vi "Daj Boze nesto.vi"() -> ()   [LabVIEW 2025]
uses:
  <vilib>/ptbypt/NI_PtbyPt.lvlib
  UARV/Timer/Timer 2013/Control Timer.ctl
panel:
  out "PumpFlag":bool
  out "SDFlag":bool
  out "error out":errorcluster
  in  "error in (no error)":errorcluster
  in  "Center":bool
  in  "Left":bool
  in  "Right":bool
  in  "Emergency off":bool
  in  "Off":bool
  in  "On":bool
  out "Stanje":string
  out "RightLED":bool
  out "LeftLED":bool
  out "CenterLED":bool
  out "Fault":bool
  out "On/Off":bool
  out "BrojacGreska":dbl
  out "Brojac":dbl
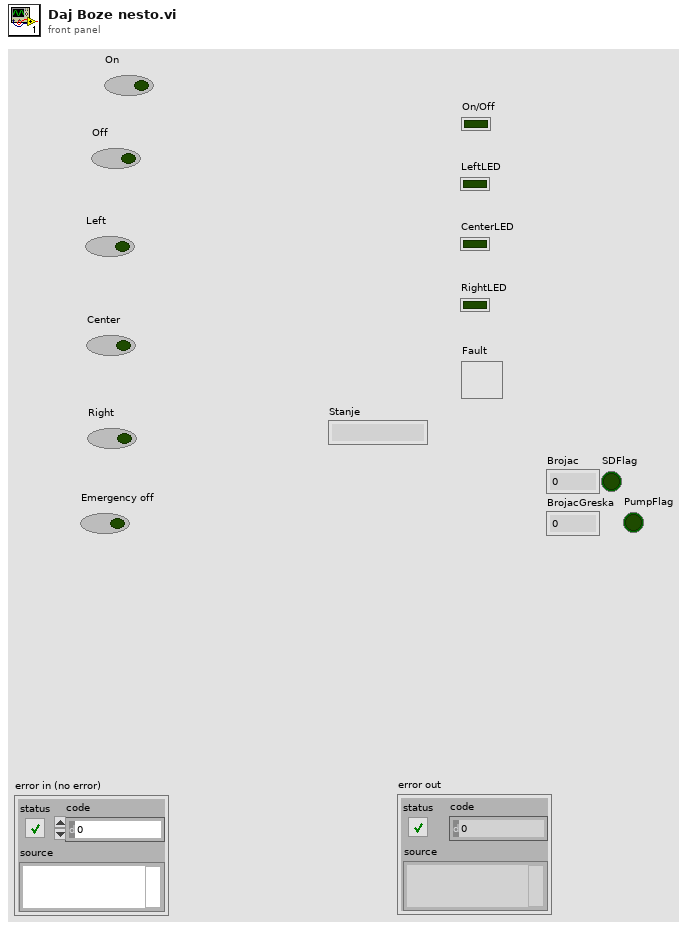
[diagram p1: front panel]
types:
  T1 = typedef "Control Timer.ctl" = enum16{"Timecheck", "Reset"}
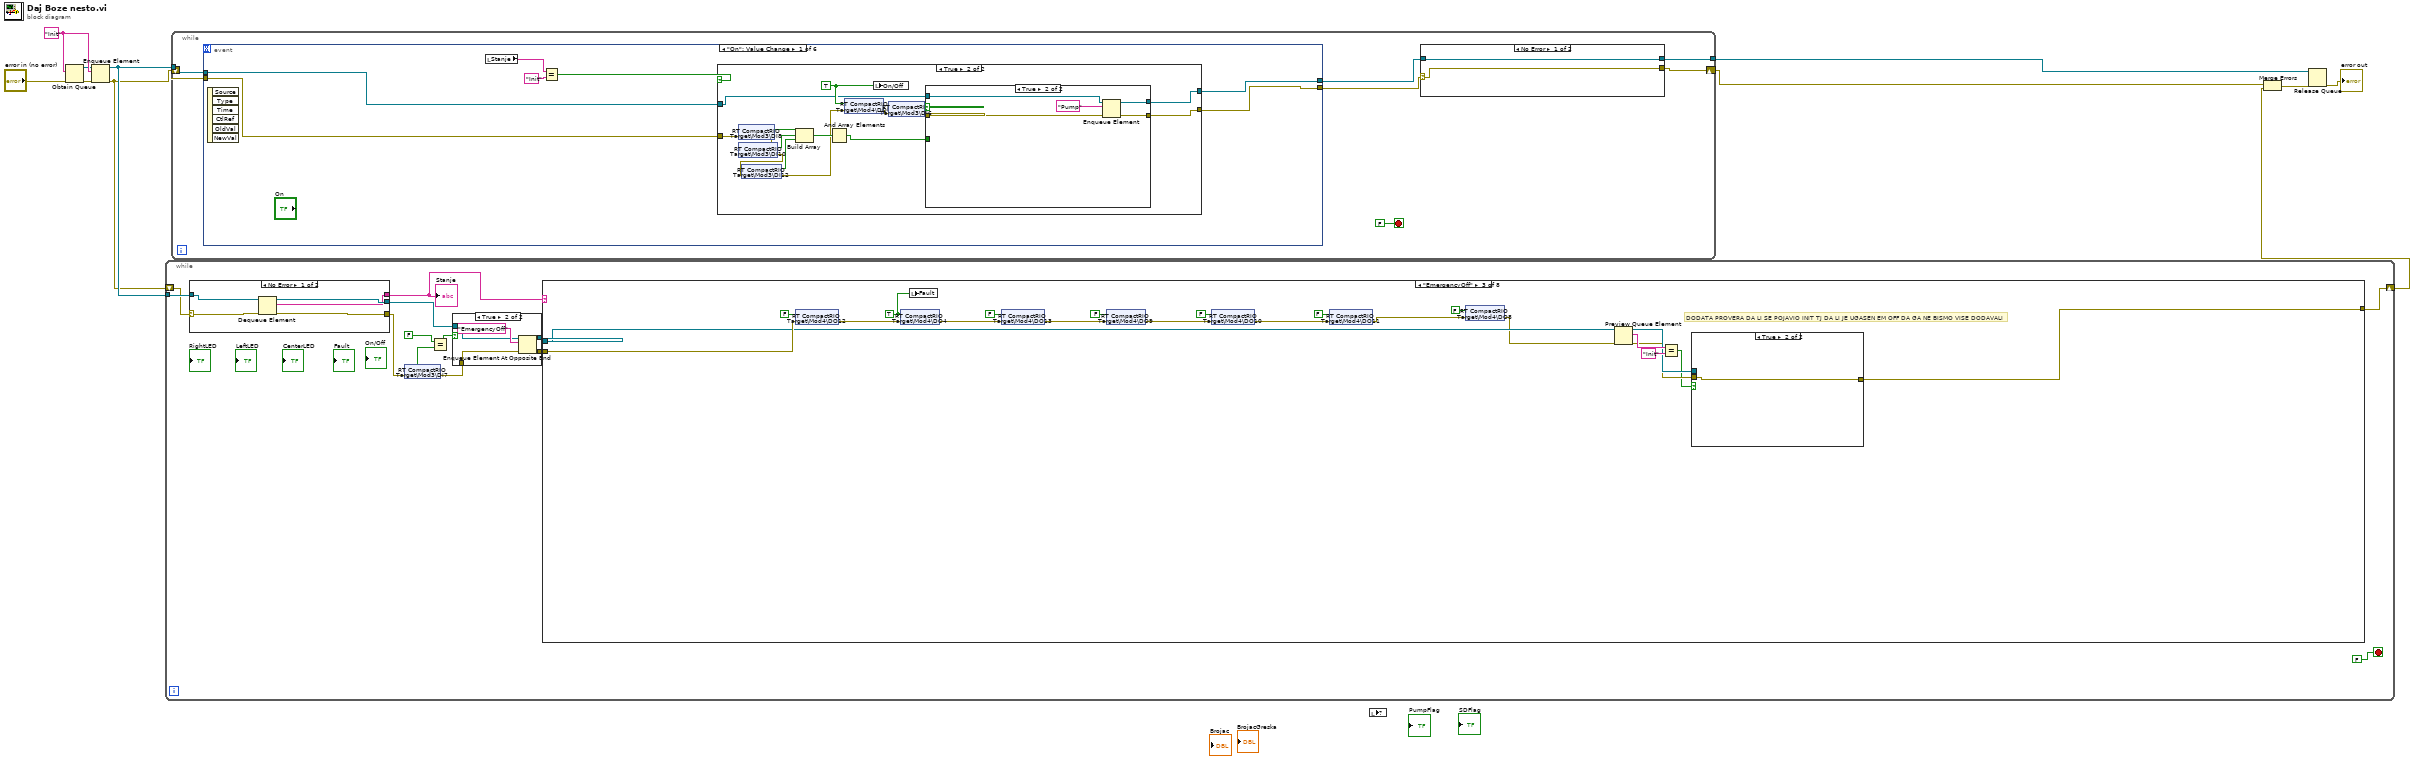
[diagram p0: block diagram]
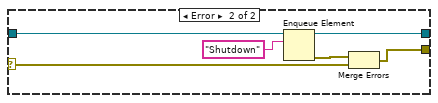
[diagram p2: hidden frame]
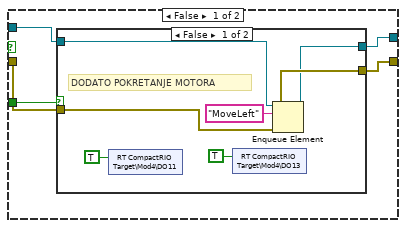
[diagram p4: hidden frame]
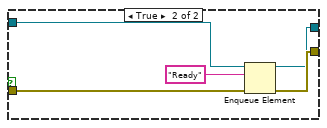
[diagram p5: hidden frame]
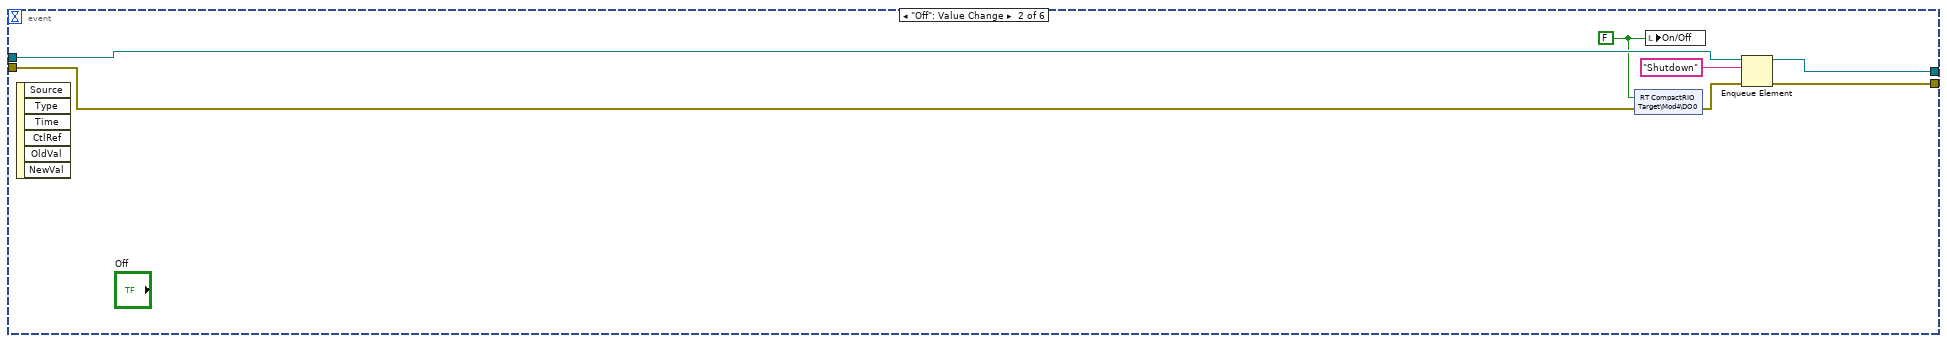
[diagram p6: hidden frame]
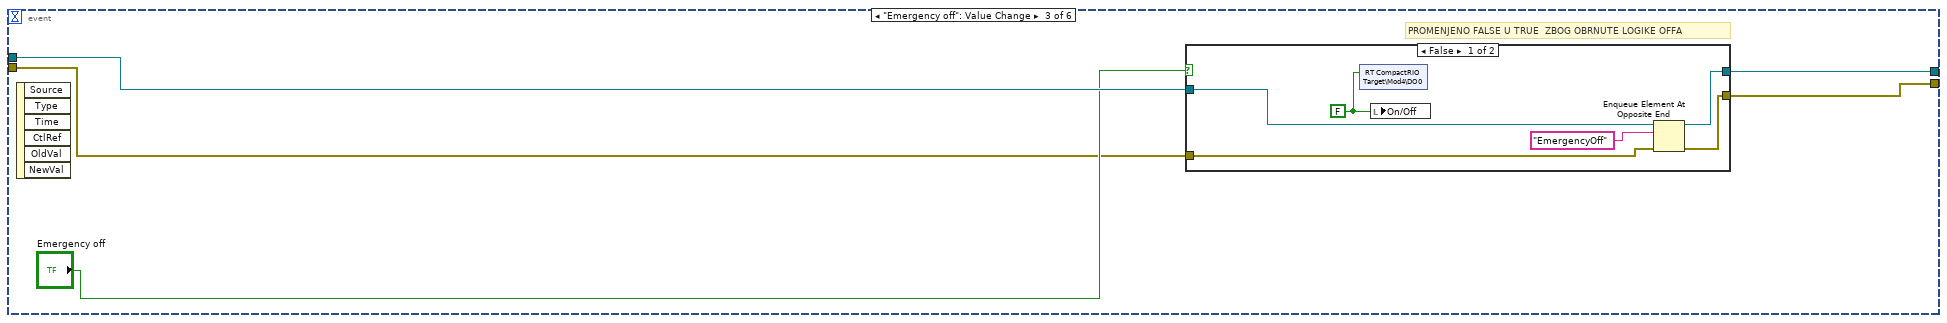
[diagram p7: hidden frame]
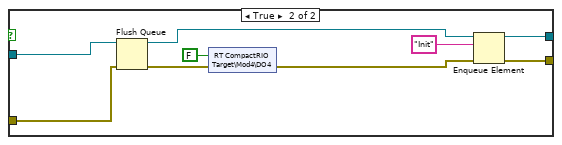
[diagram p8: hidden frame]
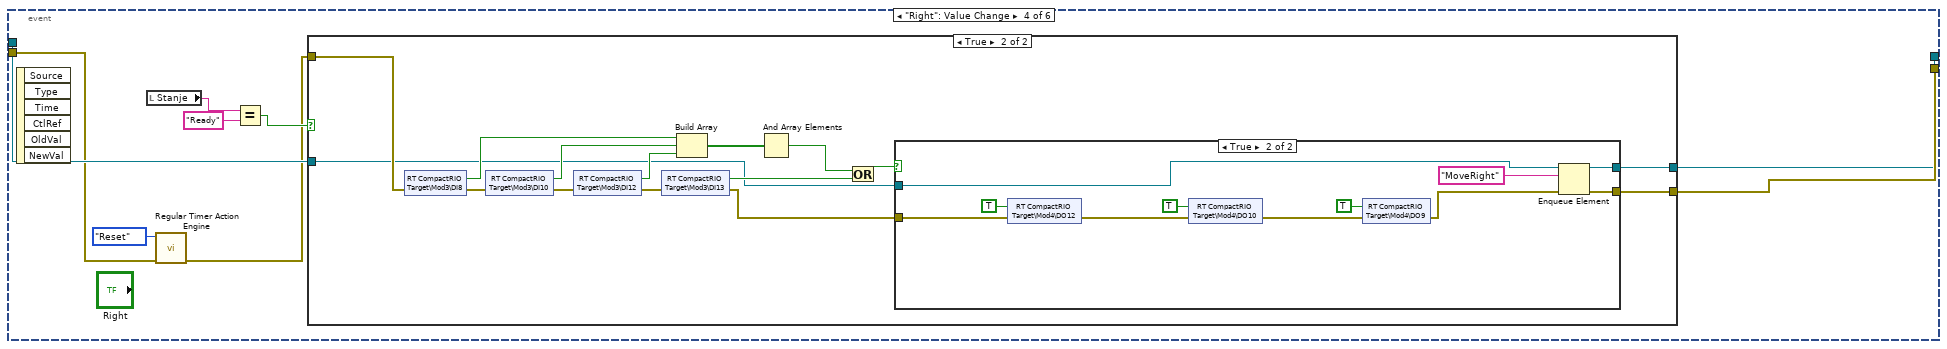
[diagram p9: hidden frame]
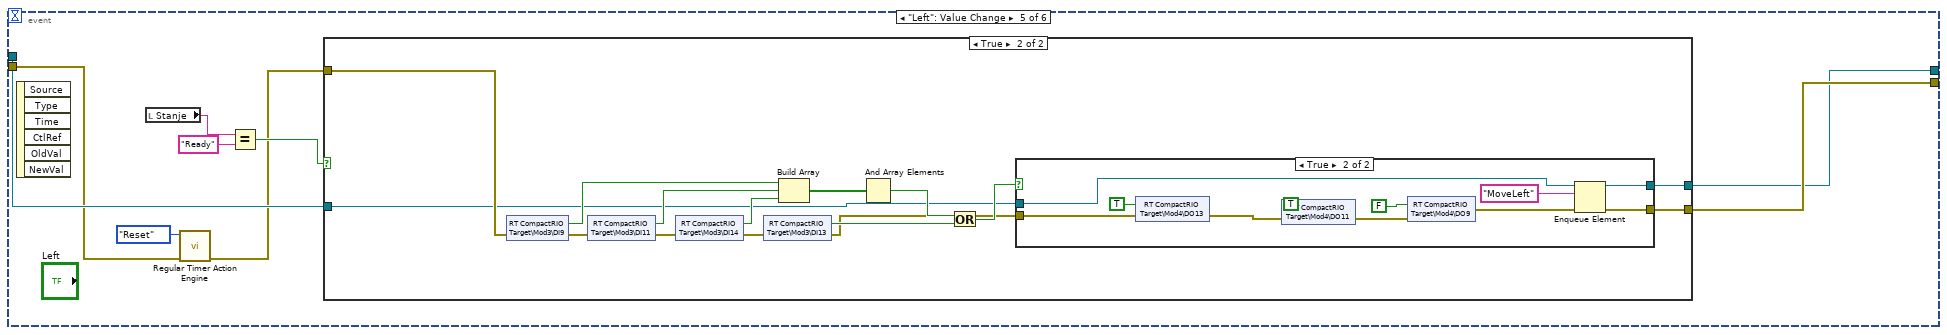
[diagram p12: hidden frame]
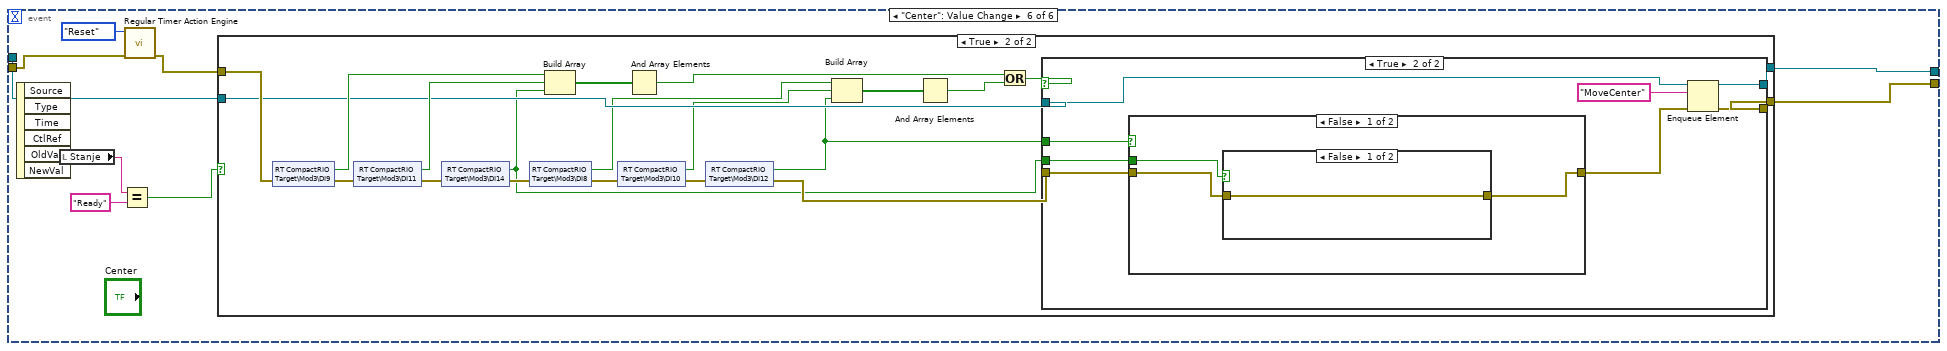
[diagram p15: hidden frame]
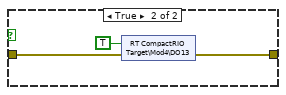
[diagram p18: hidden frame]
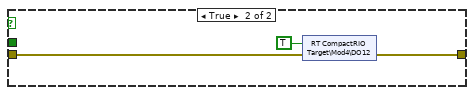
[diagram p19: hidden frame]
diagram:
  w11 = "Init"
  n1 = Obtain Queue(element data type=w11, error in (no error)="error in (no error)") -> (queue out=w9:refnum<queue>, error out=w10:errorcluster)  [unwired: 3 in, 1 out]
  n2 = Enqueue Element(queue=w9, element=w11, error in (no error)=w10) -> (queue out=w8:refnum<queue>, error out=w5:errorcluster)  [unwired: 1 in, 1 out]
  n3 = while {
    tunnel: w8 -> [w24]
    shift-right: [w12] -> w4
    shift-left: w5 -> [w13]
    stop <- FALSE stop-if-true
    n4 = case shown="No Error" w13 {
      selector: w13 -> [w567 w572]
      tunnel: w24 -> [w563 w571]
      tunnel: [w566 w570] -> w22
      tunnel: [w565 w569] -> w16
      tunnel: [w564 w568] -> w23
      frame No Error {
        n5 = Dequeue Element(queue=w563, error in (no error)=w567) -> (queue out=w565:refnum<queue>, element=w564:string, error out=w566:errorcluster)  [unwired: 1 in, 1 out]
      }
      frame Error {
        w568 = "Shutdown" ("element")
        n6 = Enqueue Element(queue=w571, element=w568, error in (no error)=w572) -> (queue out=w569:refnum<queue>, error out=w570:errorcluster)  [unwired: 1 in, 1 out]
      }
    }
    "Stanje" <- w23
    n7 = shared-variable "RT CompactRIO Target\\Mod3\\DI7"(error in=w22) -> (w21:bool, error out=w18:errorcluster)
    n8 = Equal?(x=FALSE, y=w21) -> (x = y?=w19:bool)
    n9 = case shown="True" w19 {
      tunnel: w18 -> [w26 w28]
      tunnel: [w26 w30] -> w17
      tunnel: w16 -> [w25 w27]
      tunnel: [w25 w29] -> w15
      frame False {
      }
      frame True {
        n10 = Enqueue Element At Opposite End(queue=w27, element="EmergencyOff", error in (no error)=w28) -> (queue out=w29:refnum<queue>, error out=w30:errorcluster)  [unwired: 1 in, 1 out]
      }
    }
    n11 = case shown="\"EmergencyOff\"" w23 {
      selector: w23 -> [_ _ _ _ _ _ _ w556]
      tunnel: [w43 w82 w96 w125 w148 w287 w427 w557] -> w12
      tunnel: w17 -> [w38 w86 w104 w123 w142 w281 w421 w554]
      tunnel: w15 -> [_ w81 w103 w124 w143 w282 w422 w555]
      frame "Init", Default {
        # "DOADATA REINIICILIZACIJA NOVIH PROMENLJIVIH"
        n12 = shared-variable "RT CompactRIO Target\\Mod4\\DO0"(FALSE ("DO0"), error in=w38) -> (error out=w37:errorcluster)
        n13 = shared-variable "RT CompactRIO Target\\Mod3\\DI12"(error in=w37) -> (w72:bool, error out=w70:errorcluster)
        n14 = shared-variable "RT CompactRIO Target\\Mod3\\DI10"(error in=w70) -> (w73:bool, error out=w69:errorcluster)
        n15 = shared-variable "RT CompactRIO Target\\Mod3\\DI8"(error in=w69) -> (w74:bool, error out=w59:errorcluster)
        n16 = Build Array(w74, w73, w72) -> (w71:bool[])
        n17 = And Array Elements(Boolean array=w71) -> (logical AND=w55:bool)
        n18 = local write "LeftLED"(w55) -> ()
        n19 = shared-variable "RT CompactRIO Target\\Mod4\\DO1"(w55, error in=w59) -> (error out=w58:errorcluster)
        n20 = shared-variable "RT CompactRIO Target\\Mod3\\DI14"(error in=w58) -> (w66:bool, error out=w64:errorcluster)
        n21 = shared-variable "RT CompactRIO Target\\Mod3\\DI11"(error in=w64) -> (w67:bool, error out=w63:errorcluster)
        n22 = shared-variable "RT CompactRIO Target\\Mod3\\DI9"(error in=w63) -> (w68:bool, error out=w57:errorcluster)
        n23 = Build Array(w68, w67, w66) -> (w65:bool[])
        n24 = And Array Elements(Boolean array=w65) -> (logical AND=w53:bool)
        n25 = local write "RightLED"(w53) -> ()
        n26 = shared-variable "RT CompactRIO Target\\Mod4\\DO3"(w53, error in=w57) -> (error out=w56:errorcluster)
        n27 = shared-variable "RT CompactRIO Target\\Mod3\\DI13"(error in=w56) -> (w54:bool, error out=w62:errorcluster)
        n28 = local write "Fault"(FALSE) -> ()
        n29 = local write "CenterLED"(w54) -> ()
        n30 = shared-variable "RT CompactRIO Target\\Mod4\\DO2"(w54, error in=w62) -> (error out=w51:errorcluster)
        n31 = shared-variable "RT CompactRIO Target\\Mod4\\DO4"(FALSE ("DO4"), error in=w51) -> (error out=w50:errorcluster)
        n32 = shared-variable "RT CompactRIO Target\\Mod4\\DO13"(FALSE ("DO15"), error in=w50) -> (error out=w36:errorcluster)
        n33 = shared-variable "RT CompactRIO Target\\Mod4\\DO12"(FALSE ("DO14"), error in=w36) -> (error out=w61:errorcluster)
        n34 = shared-variable "RT CompactRIO Target\\Mod4\\DO11"(FALSE ("DO13"), error in=w61) -> (error out=w42:errorcluster)
        n35 = shared-variable "RT CompactRIO Target\\Mod4\\DO8"(FALSE ("DO10"), error in=w42) -> (error out=w41:errorcluster)
        n36 = shared-variable "RT CompactRIO Target\\Mod4\\DO10"(FALSE ("DO12"), error in=w41) -> (error out=w60:errorcluster)
        n37 = shared-variable "RT CompactRIO Target\\Mod4\\DO9"(FALSE ("DO11"), error in=w60) -> (error out=w34:errorcluster)
        n38 = invoke on="SDFlag" class="Bool (strict)" method="Reinit To Default"(error in=w34) -> (error out=w33:errorcluster)  [unwired: 2 in, 2 out]
        n39 = invoke on="PumpFlag" class="Bool (strict)" method="Reinit To Default"(error in=w33) -> (error out=w32:errorcluster)  [unwired: 2 in, 2 out]
        n40 = invoke on="On/Off" class="Bool (strict)" method="Reinit To Default"(error in=w32) -> (error out=w40:errorcluster)  [unwired: 2 in, 2 out]
        n41 = invoke on="On" class="Bool (strict)" method="Reinit To Default"(error in=w40) -> (error out=w44:errorcluster)  [unwired: 2 in, 2 out]
        n42 = invoke on="Off" class="Bool (strict)" method="Reinit To Default"(error in=w44) -> (error out=w48:errorcluster)  [unwired: 2 in, 2 out]
        n43 = invoke on="Emergency off" class="Bool (strict)" method="Reinit To Default"(error in=w48) -> (error out=w47:errorcluster)  [unwired: 2 in, 2 out]
        n44 = invoke on="Right" class="Bool (strict)" method="Reinit To Default"(error in=w47) -> (error out=w46:errorcluster)  [unwired: 2 in, 2 out]
        n45 = invoke on="Left" class="Bool (strict)" method="Reinit To Default"(error in=w46) -> (error out=w45:errorcluster)  [unwired: 2 in, 2 out]
        n46 = invoke on="Center" class="Bool (strict)" method="Reinit To Default"(error in=w45) -> (error out=w43:errorcluster)  [unwired: 2 in, 2 out]
      }
      frame "Shutdown" {
        n47 = shared-variable "RT CompactRIO Target\\Mod4\\DO8"(FALSE ("DO8"), error in=w86) -> (error out=w85:errorcluster)
        n48 = shared-variable "RT CompactRIO Target\\Mod4\\DO9"(FALSE ("DO11"), error in=w85) -> (error out=w95:errorcluster)
        n49 = shared-variable "RT CompactRIO Target\\Mod4\\DO10"(FALSE ("DO12"), error in=w95) -> (error out=w87:errorcluster)
        n50 = shared-variable "RT CompactRIO Target\\Mod4\\DO11"(FALSE ("DO13"), error in=w87) -> (error out=w94:errorcluster)
        n51 = shared-variable "RT CompactRIO Target\\Mod4\\DO12"(FALSE ("DO14"), error in=w94) -> (error out=w93:errorcluster)
        n52 = shared-variable "RT CompactRIO Target\\Mod4\\DO13"(FALSE ("DO15"), error in=w93) -> (error out=w83:errorcluster)
        n53 = Enqueue Element(queue=w81, element="Init", error in (no error)=w83) -> (error out=w82:errorcluster)  [unwired: 1 in, 2 out]
      }
      frame "EmergencyOff" {
        w107 = TRUE ("DO4")
        # "DODATA PROVERA DA LI SE POJAVIO INIT TJ DA LI JE UGASEN EM OFF DA GA NE BISMO VISE DODAVALI"
        n54 = shared-variable "RT CompactRIO Target\\Mod4\\DO12"(FALSE ("DO14"), error in=w104) -> (error out=w109:errorcluster)
        n55 = shared-variable "RT CompactRIO Target\\Mod4\\DO4"(w107, error in=w109) -> (error out=w108:errorcluster)
        n56 = local write "Fault"(w107) -> ()
        n57 = shared-variable "RT CompactRIO Target\\Mod4\\DO13"(FALSE ("DO15"), error in=w108) -> (error out=w111:errorcluster)
        n58 = shared-variable "RT CompactRIO Target\\Mod4\\DO9"(FALSE ("DO11"), error in=w111) -> (error out=w117:errorcluster)
        n59 = shared-variable "RT CompactRIO Target\\Mod4\\DO10"(FALSE ("DO12"), error in=w117) -> (error out=w110:errorcluster)
        n60 = shared-variable "RT CompactRIO Target\\Mod4\\DO11"(FALSE ("DO13"), error in=w110) -> (error out=w106:errorcluster)
        n61 = shared-variable "RT CompactRIO Target\\Mod4\\DO8"(FALSE ("DO8"), error in=w106) -> (error out=w100:errorcluster)
        n62 = Preview Queue Element(queue=w103, error in (no error)=w100) -> (queue out=w99:refnum<queue>, element=w102:string, error out=w98:errorcluster)  [unwired: 1 in, 1 out]
        n63 = Equal?(x=w102, y="Init") -> (x = y?=w97:bool)
        n64 = case shown="True" w97 {
          tunnel: w99 -> [w120 _]
          tunnel: w98 -> [w119 w122]
          tunnel: [w118 w122] -> w96
          frame False {
            n65 = Enqueue Element At Opposite End(queue=w120, element="EmergencyOff", error in (no error)=w119) -> (error out=w118:errorcluster)  [unwired: 1 in, 2 out]
          }
          frame True {
          }
        }
      }
      frame "Pump" {
        n66 = shared-variable "RT CompactRIO Target\\Mod3\\DI6"(error in=w123) -> (w128:bool, error out=w126:errorcluster)
        n67 = call <vilib>:"Boolean Crossing PtByPt.vi"("direction"=enum16{"either", "false-true", "true-false"}."true-false", "input"=w128) -> ("crossing"=w127:bool)  [unwired: 1 in]
        n68 = case shown="False" w127 {
          tunnel: w126 -> [w132 w138]
          tunnel: [w135 w141] -> w125
          tunnel: w124 -> [w130 w136]
          frame False {
            n69 = shared-variable "RT CompactRIO Target\\Mod4\\DO8"(TRUE ("DO10"), error in=w132) -> (error out=w131:errorcluster)
            n70 = Enqueue Element(queue=w130, element="Pump", error in (no error)=w131) -> (error out=w135:errorcluster)  [unwired: 1 in, 2 out]
          }
          frame True {
            n71 = shared-variable "RT CompactRIO Target\\Mod4\\DO8"(FALSE ("DO10"), error in=w138) -> (error out=w137:errorcluster)
            n72 = Enqueue Element(queue=w136, element="Ready", error in (no error)=w137) -> (error out=w141:errorcluster)  [unwired: 1 in, 2 out]
          }
        }
      }
      frame "MoveRight" {
        n73 = shared-variable "RT CompactRIO Target\\Mod3\\DI6"(error in=w142) -> (w146:bool, error out=w147:errorcluster)
        n74 = call <vilib>:"Boolean Crossing PtByPt.vi"("direction"=enum16{"either", "false-true", "true-false"}."false-true", "input"=w146) -> ("crossing"=w144:bool)  [unwired: 1 in]
        n75 = case shown="False" w144 {
          tunnel: w147 -> [w178 w280]
          tunnel: [w175 w280] -> w148
          tunnel: w143 -> [w157 _]
          frame False {
            n76 = shared-variable "RT CompactRIO Target\\Mod3\\DI9"(error in=w178) -> (w182:bool, error out=w177:errorcluster)
            n77 = shared-variable "RT CompactRIO Target\\Mod3\\DI11"(error in=w177) -> (w181:bool, error out=w176:errorcluster)
            n78 = shared-variable "RT CompactRIO Target\\Mod3\\DI14"(error in=w176) -> (w180:bool, error out=w164:errorcluster)
            n79 = shared-variable "RT CompactRIO Target\\Mod3\\DI12"(error in=w164) -> (w171:bool, error out=w169:errorcluster)
            n80 = Build Array(w182, w181, w180) -> (w179:bool[])
            n81 = shared-variable "RT CompactRIO Target\\Mod3\\DI10"(error in=w169) -> (w172:bool, error out=w168:errorcluster)
            n82 = And Array Elements(Boolean array=w179) -> (logical AND=w174:bool)
            n83 = shared-variable "RT CompactRIO Target\\Mod3\\DI8"(error in=w168) -> (w173:bool, error out=w167:errorcluster)
            n84 = shared-variable "RT CompactRIO Target\\Mod3\\DI13"(error in=w167) -> (w162:bool, error out=w166:errorcluster)
            n85 = Build Array(w173, w172, w171) -> (w170:bool[])
            n86 = local write "CenterLED"(w162) -> ()
            n87 = shared-variable "RT CompactRIO Target\\Mod4\\DO2"(w162, error in=w166) -> (error out=w165:errorcluster)
            n88 = And Array Elements(Boolean array=w170) -> (logical AND=w163:bool)
            n89 = shared-variable "RT CompactRIO Target\\Mod4\\DO1"(w163, error in=w165) -> (error out=w156:errorcluster)
            n90 = local write "LeftLED"(w163) -> ()
            n91 = Preview Queue Element(queue=w157, error in (no error)=w156) -> (queue out=w154:refnum<queue>, element=w150:string, error out=w155:errorcluster)  [unwired: 1 in, 1 out]
            n92 = Equal?(x=w150, y="Shutdown") -> (x = y?=w151:bool)
            n93 = case shown="True" w151 {
              tunnel: w155 -> [w183 w188]
              tunnel: w154 -> [w184 w187]
              tunnel: [w184 w186] -> w153
              tunnel: [w183 w185] -> w152
              frame False {
              }
              frame True {
                n94 = Flush Queue(queue=w187, error in (no error)=w188) -> (queue out=w186:refnum<queue>, error out=w185:errorcluster)  [unwired: 1 out]
                n95 = local write "SDFlag"(TRUE ("SDFlag")) -> ()
              }
            }
            n96 = feedback #1() -> (w161:dbl)  [unwired: 1 in]
            n97 = feedback #2() -> (w159:dbl)  [unwired: 1 in]
            n98 = case shown="True" w174 {
              tunnel: [w198 w260] -> w175
              tunnel: w161 -> [w195 _]
              tunnel: [w194 0.0] -> w160
              tunnel: w159 -> [w193 _]
              tunnel: [w192 0.0] -> w158
              tunnel: w153 -> [w190 w251]
              tunnel: w152 -> [w191 w250]
              frame False {
                n99 = call "Regular Timer Action Engine.vi"("Enum"=Control_Timer."Timecheck", "Time Target"=0.5, "error in"=w191) -> ("Status"=w204:cluster{"Running":bool, "Done":bool}, "error out"=w201:errorcluster)  [unwired: 6 in]
                n100 = Unbundle By Name(w204) -> ("Done"=w203:bool)  [unwired: 1 out]
                n101 = feedback #3() -> (w202:bool)  [unwired: 1 in]
                n102 = case shown="True" w203 {
                  tunnel: [w212 w231] -> w197
                  tunnel: w202 -> [w212 w230]
                  tunnel: w201 -> [w211 w228]
                  tunnel: [w211 w222] -> w200
                  tunnel: w193 -> [w210 w227]
                  tunnel: [w210 w223] -> w192
                  tunnel: w195 -> [w209 w221]
                  tunnel: [w209 w218] -> w194
                  tunnel: [w208 w217] -> w196
                  tunnel: w190 -> [w208 w213]
                  frame False {
                  }
                  frame True {
                    n103 = Increment(x=w227) -> (x+1=w224:dbl)
                    n104 = Increment(x=w221) -> (x+1=w216:dbl)
                    n105 = local write "Brojac"(w224) -> ()
                    n106 = local write "BrojacGreska"(w216) -> ()
                    n107 = Not(x=w230) -> (.not. x?=w231:bool)
                    n108 = Equal?(x=w216, y=30.0) -> (x = y?=w219:bool)
                    n109 = Equal?(x=4.0, y=w224) -> (x = y?=w226:bool)
                    n110 = call "Regular Timer Action Engine.vi"("Enum"=Control_Timer."Reset", "error in"=w228) -> ("error out"=w215:errorcluster)  [unwired: 7 in, 1 out]
                    n111 = case shown="True" w219 {
                      tunnel: [w234 0.0] -> w218
                      tunnel: w216 -> [w234 _]
                      tunnel: [w232 w238] -> w217
                      tunnel: w215 -> [w233 w237]
                      tunnel: [w233 w236] -> w214
                      tunnel: w213 -> [w232 w235]
                      frame False {
                      }
                      frame True {
                        n112 = Flush Queue(queue=w235, error in (no error)=w237) -> (queue out=w240:refnum<queue>, error out=w241:errorcluster)  [unwired: 1 out]
                        n113 = Enqueue Element At Opposite End(queue=w240, element="EmergencyOff", error in (no error)=w241) -> (queue out=w238:refnum<queue>, error out=w236:errorcluster)  [unwired: 1 in, 1 out]
                      }
                    }
                    n114 = case shown="True" w226 {
                      tunnel: w224 -> [w244 _]
                      tunnel: [w244 0.0] -> w223
                      tunnel: [w243 w245] -> w222
                      tunnel: w214 -> [w243 w245]
                      frame False {
                      }
                      frame True {
                        n115 = shared-variable "RT CompactRIO Target\\Mod4\\DO10"(FALSE ("DO12")) -> ()  [unwired: 1 in, 1 out]
                      }
                    }
                  }
                }
                n116 = feedback-in #3(w197) -> ()
                n117 = local write "RightLED"(w197) -> ()
                n118 = shared-variable "RT CompactRIO Target\\Mod4\\DO3"(w197, error in=w200) -> (error out=w199:errorcluster)
                n119 = Enqueue Element(queue=w196, element="MoveRight", error in (no error)=w199) -> (error out=w198:errorcluster)  [unwired: 1 in, 2 out]
              }
              frame True {
                w254 = TRUE ("DO3")
                # "DODATA OBRADA PUMP FLAGA AKO NIJE SD FLAG"
                n120 = shared-variable "RT CompactRIO Target\\Mod4\\DO12"(FALSE ("DO15"), error in=w250) -> (error out=w257:errorcluster)
                n121 = shared-variable "RT CompactRIO Target\\Mod4\\DO10"(FALSE ("DO13"), error in=w257) -> (error out=w256:errorcluster)
                n122 = local write "RightLED"(w254) -> ()
                n123 = shared-variable "RT CompactRIO Target\\Mod4\\DO3"(w254, error in=w256) -> (error out=w255:errorcluster)
                n124 = local read "SDFlag"() -> (w249:bool)
                n125 = local read "PumpFlag"() -> (w248:bool)
                n126 = case shown="False" w249 {
                  tunnel: [w264 w278] -> w260
                  tunnel: w255 -> [w263 w274]
                  tunnel: w251 -> [w262 w275]
                  tunnel: w248 -> [w261 _]
                  frame False {
                    n127 = case shown="True" w261 {
                      tunnel: [w267 w271] -> w264
                      tunnel: w263 -> [w266 w272]
                      tunnel: w262 -> [w265 w273]
                      frame False {
                        n128 = Enqueue Element(queue=w265, element="Ready", error in (no error)=w266) -> (error out=w267:errorcluster)  [unwired: 1 in, 2 out]
                      }
                      frame True {
                        n129 = local write "PumpFlag"(FALSE ("PumpFlag")) -> ()
                        n130 = Enqueue Element(queue=w273, element="Pump", error in (no error)=w272) -> (error out=w271:errorcluster)  [unwired: 1 in, 2 out]
                      }
                    }
                  }
                  frame True {
                    n131 = local write "SDFlag"(FALSE ("SDFlag")) -> ()
                    n132 = Enqueue Element(queue=w275, element="Shutdown", error in (no error)=w274) -> (error out=w278:errorcluster)  [unwired: 1 in, 2 out]
                  }
                }
              }
            }
            n133 = feedback-in #1(w160) -> ()
            n134 = feedback-in #2(w158) -> ()
          }
          frame True {
            # "DODAT FALG UMESTO POKRETANJA PUMPE ODMAH"
            n135 = local write "PumpFlag"(TRUE ("PumpFlag")) -> ()
          }
        }
      }
      frame "MoveLeft" {
        n136 = shared-variable "RT CompactRIO Target\\Mod3\\DI6"(error in=w281) -> (w286:bool, error out=w284:errorcluster)
        n137 = call <vilib>:"Boolean Crossing PtByPt.vi"("direction"=enum16{"either", "false-true", "true-false"}."false-true", "input"=w286) -> ("crossing"=w283:bool)  [unwired: 1 in]
        n138 = case shown="False" w283 {
          tunnel: w284 -> [w316 w419]
          tunnel: [w313 w419] -> w287
          tunnel: w282 -> [w289 _]
          frame False {
            n139 = shared-variable "RT CompactRIO Target\\Mod3\\DI8"(error in=w316) -> (w321:bool, error out=w315:errorcluster)
            n140 = shared-variable "RT CompactRIO Target\\Mod3\\DI10"(error in=w315) -> (w320:bool, error out=w314:errorcluster)
            n141 = shared-variable "RT CompactRIO Target\\Mod3\\DI12"(error in=w314) -> (w319:bool, error out=w308:errorcluster)
            n142 = shared-variable "RT CompactRIO Target\\Mod3\\DI14"(error in=w308) -> (w310:bool, error out=w307:errorcluster)
            n143 = Build Array(w321, w320, w319) -> (w318:bool[])
            n144 = shared-variable "RT CompactRIO Target\\Mod3\\DI11"(error in=w307) -> (w311:bool, error out=w306:errorcluster)
            n145 = And Array Elements(Boolean array=w318) -> (logical AND=w317:bool)
            n146 = shared-variable "RT CompactRIO Target\\Mod3\\DI9"(error in=w306) -> (w312:bool, error out=w305:errorcluster)
            n147 = shared-variable "RT CompactRIO Target\\Mod3\\DI13"(error in=w305) -> (w301:bool, error out=w304:errorcluster)
            n148 = Build Array(w312, w311, w310) -> (w309:bool[])
            n149 = shared-variable "RT CompactRIO Target\\Mod4\\DO2"(w301, error in=w304) -> (error out=w303:errorcluster)
            n150 = local write "CenterLED"(w301) -> ()
            n151 = And Array Elements(Boolean array=w309) -> (logical AND=w302:bool)
            n152 = local write "RightLED"(w302) -> ()
            n153 = shared-variable "RT CompactRIO Target\\Mod4\\DO3"(w302, error in=w303) -> (error out=w296:errorcluster)
            n154 = Preview Queue Element(queue=w289, error in (no error)=w296) -> (queue out=w292:refnum<queue>, element=w295:string, error out=w291:errorcluster)  [unwired: 1 in, 1 out]
            n155 = Equal?(x=w295, y="Shutdown") -> (x = y?=w293:bool)
            n156 = case shown="True" w293 {
              tunnel: w292 -> [w322 w328]
              tunnel: w291 -> [w323 w327]
              tunnel: [w323 w326] -> w290
              tunnel: [w322 w324] -> w288
              frame False {
              }
              frame True {
                n157 = Flush Queue(queue=w328, error in (no error)=w327) -> (queue out=w324:refnum<queue>, error out=w326:errorcluster)  [unwired: 1 out]
                n158 = local write "SDFlag"(TRUE ("SDFlag")) -> ()
              }
            }
            n159 = feedback #4() -> (w300:dbl)  [unwired: 1 in]
            n160 = feedback #5() -> (w298:dbl)  [unwired: 1 in]
            n161 = case shown="True" w317 {
              tunnel: w290 -> [w333 w396]
              tunnel: [w346 w400] -> w313
              tunnel: w288 -> [w336 w392]
              tunnel: w300 -> [w332 _]
              tunnel: [w331 0.0] -> w299
              tunnel: w298 -> [w330 _]
              tunnel: [w329 0.0] -> w297
              frame False {
                n162 = call "Regular Timer Action Engine.vi"("Enum"=Control_Timer."Timecheck", "Time Target"=0.5, "error in"=w333) -> ("Status"=w342:cluster{"Running":bool, "Done":bool}, "error out"=w339:errorcluster)  [unwired: 6 in]
                n163 = Unbundle By Name(w342) -> ("Done"=w341:bool)  [unwired: 1 out]
                n164 = feedback #6() -> (w340:bool)  [unwired: 1 in]
                n165 = case shown="True" w341 {
                  tunnel: [w351 w370] -> w337
                  tunnel: w340 -> [w351 w369]
                  tunnel: w339 -> [w350 w358]
                  tunnel: [w350 w367] -> w334
                  tunnel: [w349 w363] -> w329
                  tunnel: w330 -> [w349 w366]
                  tunnel: w332 -> [w348 w354]
                  tunnel: w336 -> [w347 w360]
                  tunnel: [w347 w359] -> w335
                  tunnel: [w348 w355] -> w331
                  frame False {
                  }
                  frame True {
                    n166 = Increment(x=w366) -> (x+1=w353:dbl)
                    n167 = local write "Brojac"(w353) -> ()
                    n168 = Increment(x=w354) -> (x+1=w352:dbl)
                    n169 = local write "BrojacGreska"(w352) -> ()
                    n170 = Equal?(x=w352, y=30.0) -> (x = y?=w361:bool)
                    n171 = Equal?(x=w353, y=4.0) -> (x = y?=w364:bool)
                    n172 = Not(x=w369) -> (.not. x?=w370:bool)
                    n173 = case shown="True" w364 {
                      tunnel: w353 -> [w383 _]
                      tunnel: [w383 0.0] -> w363
                      tunnel: w358 -> [w382 w385]
                      tunnel: [w382 w384] -> w357
                      frame False {
                      }
                      frame True {
                        n174 = shared-variable "RT CompactRIO Target\\Mod4\\DO11"(FALSE ("DO13"), error in=w385) -> (error out=w384:errorcluster)
                      }
                    }
                    n175 = case shown="True" w361 {
                      tunnel: w352 -> [w373 _]
                      tunnel: [w373 0.0] -> w355
                      tunnel: w360 -> [w372 w380]
                      tunnel: [w372 w378] -> w359
                      tunnel: w357 -> [w371 w377]
                      tunnel: [w371 w375] -> w356
                      frame False {
                      }
                      frame True {
                        n176 = Flush Queue(queue=w380, error in (no error)=w377) -> (queue out=w379:refnum<queue>, error out=w376:errorcluster)  [unwired: 1 out]
                        n177 = Enqueue Element At Opposite End(queue=w379, element="EmergencyOff", error in (no error)=w376) -> (queue out=w378:refnum<queue>, error out=w375:errorcluster)  [unwired: 1 in, 1 out]
                      }
                    }
                    n178 = call "Regular Timer Action Engine.vi"("Enum"=Control_Timer."Reset", "error in"=w356) -> ("error out"=w367:errorcluster)  [unwired: 7 in, 1 out]
                  }
                }
                n179 = feedback-in #6(w337) -> ()
                n180 = local write "LeftLED"(w337) -> ()
                n181 = shared-variable "RT CompactRIO Target\\Mod4\\DO1"(w337, error in=w334) -> (error out=w338:errorcluster)
                n182 = Enqueue Element(queue=w335, element="MoveLeft", error in (no error)=w338) -> (error out=w346:errorcluster)  [unwired: 1 in, 2 out]
              }
              frame True {
                w394 = TRUE ("DO1")
                # "DODATA OBRADA PUMP FLAGA AKO NIJE SD FLAG"
                n183 = local write "LeftLED"(w394) -> ()
                n184 = shared-variable "RT CompactRIO Target\\Mod4\\DO1"(w394, error in=w396) -> (error out=w395:errorcluster)
                n185 = shared-variable "RT CompactRIO Target\\Mod4\\DO13"(FALSE ("DO15"), error in=w395) -> (error out=w397:errorcluster)
                n186 = local read "SDFlag"() -> (w389:bool)
                n187 = local read "PumpFlag"() -> (w388:bool)
                n188 = shared-variable "RT CompactRIO Target\\Mod4\\DO11"(FALSE ("DO13"), error in=w397) -> (error out=w393:errorcluster)
                n189 = case shown="False" w389 {
                  tunnel: [w404 w416] -> w400
                  tunnel: w393 -> [w403 w418]
                  tunnel: w392 -> [w402 w417]
                  tunnel: w388 -> [w401 _]
                  frame False {
                    n190 = case shown="True" w401 {
                      tunnel: [w407 w411] -> w404
                      tunnel: w403 -> [w406 w413]
                      tunnel: w402 -> [w405 w412]
                      frame False {
                        n191 = Enqueue Element(queue=w405, element="Ready", error in (no error)=w406) -> (error out=w407:errorcluster)  [unwired: 1 in, 2 out]
                      }
                      frame True {
                        n192 = local write "PumpFlag"(FALSE ("PumpFlag")) -> ()
                        n193 = Enqueue Element(queue=w412, element="Pump", error in (no error)=w413) -> (error out=w411:errorcluster)  [unwired: 1 in, 2 out]
                      }
                    }
                  }
                  frame True {
                    n194 = Enqueue Element(queue=w417, element="Shutdown", error in (no error)=w418) -> (error out=w416:errorcluster)  [unwired: 1 in, 2 out]
                    n195 = local write "SDFlag"(FALSE ("SDFlag")) -> ()
                  }
                }
              }
            }
            n196 = feedback-in #4(w299) -> ()
            n197 = feedback-in #5(w297) -> ()
          }
          frame True {
            # "DODAT FALG UMESTO POKRETANJA PUMPE ODMAH"
            n198 = local write "PumpFlag"(TRUE ("PumpFlag")) -> ()
          }
        }
      }
      frame "MoveCenter" {
        n199 = shared-variable "RT CompactRIO Target\\Mod3\\DI6"(error in=w421) -> (w426:bool, error out=w423:errorcluster)
        n200 = call <vilib>:"Boolean Crossing PtByPt.vi"("direction"=enum16{"either", "false-true", "true-false"}."false-true", "input"=w426) -> ("crossing"=w424:bool)  [unwired: 1 in]
        n201 = case shown="False" w424 {
          tunnel: [w459 w541] -> w427
          tunnel: w423 -> [w445 w541]
          tunnel: w422 -> [w435 _]
          frame False {
            n202 = shared-variable "RT CompactRIO Target\\Mod3\\DI12"(error in=w445) -> (w455:bool, error out=w453:errorcluster)
            n203 = shared-variable "RT CompactRIO Target\\Mod3\\DI10"(error in=w453) -> (w456:bool, error out=w452:errorcluster)
            n204 = shared-variable "RT CompactRIO Target\\Mod3\\DI8"(error in=w452) -> (w457:bool, error out=w444:errorcluster)
            n205 = shared-variable "RT CompactRIO Target\\Mod3\\DI14"(error in=w444) -> (w449:bool, error out=w447:errorcluster)
            n206 = Build Array(w457, w456, w455) -> (w454:bool[])
            n207 = shared-variable "RT CompactRIO Target\\Mod3\\DI11"(error in=w447) -> (w450:bool, error out=w446:errorcluster)
            n208 = And Array Elements(Boolean array=w454) -> (logical AND=w439:bool)
            n209 = shared-variable "RT CompactRIO Target\\Mod3\\DI9"(error in=w446) -> (w451:bool, error out=w443:errorcluster)
            n210 = local write "LeftLED"(w439) -> ()
            n211 = shared-variable "RT CompactRIO Target\\Mod4\\DO1"(w439, error in=w443) -> (error out=w442:errorcluster)
            n212 = Build Array(w451, w450, w449) -> (w448:bool[])
            n213 = And Array Elements(Boolean array=w448) -> (logical AND=w440:bool)
            n214 = local write "RightLED"(w440) -> ()
            n215 = shared-variable "RT CompactRIO Target\\Mod4\\DO3"(w440, error in=w442) -> (error out=w441:errorcluster)
            n216 = shared-variable "RT CompactRIO Target\\Mod3\\DI13"(error in=w441) -> (w458:bool, error out=w436:errorcluster)
            n217 = Preview Queue Element(queue=w435, error in (no error)=w436) -> (queue out=w431:refnum<queue>, element=w434:string, error out=w430:errorcluster)  [unwired: 1 in, 1 out]
            n218 = Equal?(x=w434, y="Shutdown") -> (x = y?=w432:bool)
            n219 = case shown="True" w432 {
              tunnel: w431 -> [w461 w466]
              tunnel: w430 -> [w460 w465]
              tunnel: [w460 w464] -> w429
              tunnel: [w461 w462] -> w428
              frame False {
              }
              frame True {
                n220 = local write "SDFlag"(TRUE ("SDFlag")) -> ()
                n221 = Flush Queue(queue=w466, error in (no error)=w465) -> (queue out=w462:refnum<queue>, error out=w464:errorcluster)  [unwired: 1 out]
              }
            }
            n222 = feedback #7() -> (w438:dbl)  [unwired: 1 in]
            n223 = case shown="True" w458 {
              tunnel: [w474 w522] -> w459
              tunnel: w429 -> [w475 w520]
              tunnel: w428 -> [w470 w515]
              tunnel: [w468 0.0] -> w437
              tunnel: w438 -> [w467 _]
              frame False {
                n224 = call "Regular Timer Action Engine.vi"("Enum"=Control_Timer."Timecheck", "Time Target"=0.5, "error in"=w475) -> ("Status"=w479:cluster{"Running":bool, "Done":bool}, "error out"=w476:errorcluster)  [unwired: 6 in]
                n225 = Unbundle By Name(w479) -> ("Done"=w478:bool)  [unwired: 1 out]
                n226 = feedback #8() -> (w477:bool)  [unwired: 1 in]
                n227 = case shown="False" w478 {
                  tunnel: [w486 w499] -> w471
                  tunnel: w477 -> [w486 w498]
                  tunnel: w476 -> [w485 w490]
                  tunnel: [w485 w496] -> w473
                  tunnel: w470 -> [w484 w492]
                  tunnel: [w484 w491] -> w469
                  tunnel: [w483 w488] -> w468
                  tunnel: w467 -> [w483 w487]
                  frame False {
                  }
                  frame True {
                    n228 = Increment(x=w487) -> (x+1=w493:dbl)
                    n229 = local write "BrojacGreska"(w493) -> ()
                    n230 = Equal?(x=w493, y=30.0) -> (x = y?=w494:bool)
                    n231 = case shown="True" w494 {
                      tunnel: [w502 0.0] -> w488
                      tunnel: w493 -> [w502 _]
                      tunnel: w492 -> [w500 w508]
                      tunnel: [w500 w506] -> w491
                      tunnel: w490 -> [w501 w505]
                      tunnel: [w501 w503] -> w489
                      frame False {
                      }
                      frame True {
                        n232 = Flush Queue(queue=w508, error in (no error)=w505) -> (queue out=w507:refnum<queue>, error out=w504:errorcluster)  [unwired: 1 out]
                        n233 = Enqueue Element At Opposite End(queue=w507, element="EmergencyOff", error in (no error)=w504) -> (queue out=w506:refnum<queue>, error out=w503:errorcluster)  [unwired: 1 in, 1 out]
                      }
                    }
                    n234 = Not(x=w498) -> (.not. x?=w499:bool)
                    n235 = call "Regular Timer Action Engine.vi"("Enum"=Control_Timer."Reset", "error in"=w489) -> ("error out"=w496:errorcluster)  [unwired: 7 in, 1 out]
                  }
                }
                n236 = feedback-in #8(w471) -> ()
                n237 = local write "CenterLED"(w471) -> ()
                n238 = shared-variable "RT CompactRIO Target\\Mod4\\DO2"(w471, error in=w473) -> (error out=w472:errorcluster)
                n239 = Enqueue Element(queue=w469, element="MoveCenter", error in (no error)=w472) -> (error out=w474:errorcluster)  [unwired: 1 in, 2 out]
              }
              frame True {
                w516 = TRUE ("DO2")
                # "DODATA OBRADA PUMP FLAGA AKO NIJE SD FLAG"
                n240 = shared-variable "RT CompactRIO Target\\Mod4\\DO13"(FALSE ("DO15"), error in=w520) -> (error out=w519:errorcluster)
                n241 = shared-variable "RT CompactRIO Target\\Mod4\\DO12"(FALSE ("DO14"), error in=w519) -> (error out=w518:errorcluster)
                n242 = local write "CenterLED"(w516) -> ()
                n243 = shared-variable "RT CompactRIO Target\\Mod4\\DO2"(w516, error in=w518) -> (error out=w517:errorcluster)
                n244 = local read "SDFlag"() -> (w512:bool)
                n245 = local read "PumpFlag"() -> (w511:bool)
                n246 = case shown="False" w512 {
                  tunnel: [w526 w538] -> w522
                  tunnel: w517 -> [w525 w540]
                  tunnel: w515 -> [w524 w539]
                  tunnel: w511 -> [w523 _]
                  frame False {
                    n247 = case shown="True" w523 {
                      tunnel: [w529 w533] -> w526
                      tunnel: w525 -> [w528 w535]
                      tunnel: w524 -> [w527 w534]
                      frame False {
                        n248 = Enqueue Element(queue=w527, element="Ready", error in (no error)=w528) -> (error out=w529:errorcluster)  [unwired: 1 in, 2 out]
                      }
                      frame True {
                        n249 = local write "PumpFlag"(FALSE ("PumpFlag")) -> ()
                        n250 = Enqueue Element(queue=w534, element="Pump", error in (no error)=w535) -> (error out=w533:errorcluster)  [unwired: 1 in, 2 out]
                      }
                    }
                  }
                  frame True {
                    n251 = local write "SDFlag"(FALSE ("SDFlag")) -> ()
                    n252 = Enqueue Element(queue=w539, element="Shutdown", error in (no error)=w540) -> (error out=w538:errorcluster)  [unwired: 1 in, 2 out]
                  }
                }
              }
            }
            n253 = feedback-in #7(w437) -> ()
          }
          frame True {
            # "DODAT FALG UMESTO POKRETANJA PUMPE ODMAH"
            n254 = local write "PumpFlag"(TRUE ("PumpFlag")) -> ()
          }
        }
      }
      frame "Ready" {
        n255 = Preview Queue Element(queue=w555, error in (no error)=w554) -> (queue out=w553:refnum<queue>, element=w550:string, error out=w552:errorcluster)  [unwired: 1 in, 1 out]
        n256 = Equal?(x=w550, y="MoveRight") -> (x = y?=w547:bool)
        n257 = Equal?(x=w550, y="MoveLeft") -> (x = y?=w546:bool)
        n258 = Equal?(x=w550, y="MoveCenter") -> (x = y?=w544:bool)
        n259 = Or(x=w547, y=w546) -> (x .or. y?=w545:bool)
        n260 = Or(x=w545, y=w544) -> (x .or. y?=w543:bool)
        n261 = case shown="False" w543 {
          tunnel: [w561 w562] -> w557
          tunnel: w556 -> [w560 _]
          tunnel: w553 -> [w559 _]
          tunnel: w552 -> [w558 w562]
          frame False {
            n262 = Enqueue Element(queue=w559, element=w560, error in (no error)=w558) -> (error out=w561:errorcluster)  [unwired: 1 in, 2 out]
          }
          frame True {
          }
        }
      }
    }
  }
  n263 = while {
    tunnel: w8 -> [w579]
    tunnel: [w576] -> w6
    shift-right: [w574] -> w3
    shift-left: w5 -> [w573]
    stop <- FALSE stop-if-true
    n264 = event shown="[0] \"On\": Value Change" {
      selector: _ -> [_ _ _ _ _ _]
      dyn-events: _ -> [_ _ _ _ _ _]
      timeout: _ -> [_ _ _ _ _ _]
      tunnel: w579 -> [w589 w640 w646 w668 w707 w746]
      tunnel: [w594 w639 w645 w670 w709 w748] -> w578
      tunnel: [w593 w638 w644 w669 w708 w747] -> w577
      tunnel: w573 -> [w588 w635 w642 w662 w701 w740]
      event "On": Value Change {
        n265 = event-data() -> ()  [unwired: 1 in, 6 out]
        n266 = local read "Stanje"() -> (w590:string)
        n267 = Equal?(x=w590, y="Init") -> (x = y?=w591:bool)
        n268 = case shown="True" w591 {
          tunnel: [w595 w612] -> w594
          tunnel: [w596 w611] -> w593
          tunnel: w589 -> [w596 w598]
          tunnel: w588 -> [w595 w597]
          frame False {
          }
          frame True {
            w599 = TRUE
            n269 = shared-variable "RT CompactRIO Target\\Mod3\\DI8"(error in=w597) -> (w605:bool, error out=w602:errorcluster)
            n270 = shared-variable "RT CompactRIO Target\\Mod3\\DI10"(error in=w602) -> (w606:bool, error out=w601:errorcluster)
            n271 = shared-variable "RT CompactRIO Target\\Mod3\\DI12"(error in=w601) -> (w607:bool, error out=w600:errorcluster)
            n272 = Build Array(w605, w606, w607) -> (w604:bool[])
            n273 = And Array Elements(Boolean array=w604) -> (logical AND=w603:bool)
            n274 = shared-variable "RT CompactRIO Target\\Mod4\\DO0"(w599, error in=w600) -> (error out=w608:errorcluster)
            n275 = local write "On/Off"(w599) -> ()
            n276 = shared-variable "RT CompactRIO Target\\Mod3\\DI6"(error in=w608) -> (w610:bool, error out=w609:errorcluster)
            n277 = case shown="True" w610 {
              tunnel: [w617 w633] -> w612
              tunnel: [w616 w632] -> w611
              tunnel: w609 -> [w615 w631]
              tunnel: w603 -> [w614 _]
              tunnel: w598 -> [w613 w630]
              frame False {
                n278 = case shown="False" w614 {
                  tunnel: [w623 w629] -> w617
                  tunnel: [w622 w627] -> w616
                  tunnel: w615 -> [w624 w626]
                  tunnel: w613 -> [w620 w625]
                  frame False {
                    # "DODATO POKRETANJE MOTORA"
                    n279 = shared-variable "RT CompactRIO Target\\Mod4\\DO11"(TRUE ("DO11")) -> ()  [unwired: 1 in, 1 out]
                    n280 = shared-variable "RT CompactRIO Target\\Mod4\\DO13"(TRUE ("DO13")) -> ()  [unwired: 1 in, 1 out]
                    n281 = Enqueue Element(queue=w620, element="MoveLeft", error in (no error)=w624) -> (queue out=w622:refnum<queue>, error out=w623:errorcluster)  [unwired: 1 in, 1 out]
                  }
                  frame True {
                    n282 = Enqueue Element(queue=w625, element="Ready", error in (no error)=w626) -> (queue out=w627:refnum<queue>, error out=w629:errorcluster)  [unwired: 1 in, 1 out]
                  }
                }
              }
              frame True {
                n283 = Enqueue Element(queue=w630, element="Pump", error in (no error)=w631) -> (queue out=w632:refnum<queue>, error out=w633:errorcluster)  [unwired: 1 in, 1 out]
              }
            }
          }
        }
      }
      event "Off": Value Change {
        w636 = FALSE
        n284 = event-data() -> ()  [unwired: 1 in, 6 out]
        n285 = shared-variable "RT CompactRIO Target\\Mod4\\DO0"(w636, error in=w635) -> (error out=w637:errorcluster)
        n286 = local write "On/Off"(w636) -> ()
        n287 = Enqueue Element(queue=w640, element="Shutdown", error in (no error)=w637) -> (queue out=w638:refnum<queue>, error out=w639:errorcluster)  [unwired: 1 in, 1 out]
      }
      event "Emergency off": Value Change {
        # "PROMENJENO FALSE U TRUE  ZBOG OBRNUTE LOGIKE OFFA"
        n288 = event-data() -> ()  [unwired: 1 in, 6 out]
        n289 = case shown="False" "Emergency off" {
          tunnel: w646 -> [w651 w661]
          tunnel: [w650 w660] -> w645
          tunnel: [w649 w659] -> w644
          tunnel: w642 -> [w647 w653]
          frame False {
            w648 = FALSE
            n290 = shared-variable "RT CompactRIO Target\\Mod4\\DO0"(w648) -> ()  [unwired: 1 in, 1 out]
            n291 = local write "On/Off"(w648) -> ()
            n292 = Enqueue Element At Opposite End(queue=w651, element="EmergencyOff", error in (no error)=w647) -> (queue out=w649:refnum<queue>, error out=w650:errorcluster)  [unwired: 1 in, 1 out]
          }
          frame True {
            n293 = Flush Queue(queue=w661, error in (no error)=w653) -> (queue out=w658:refnum<queue>, error out=w655:errorcluster)  [unwired: 1 out]
            n294 = shared-variable "RT CompactRIO Target\\Mod4\\DO4"(FALSE ("DO4"), error in=w655) -> (error out=w654:errorcluster)
            n295 = Enqueue Element(queue=w658, element="Init", error in (no error)=w654) -> (queue out=w659:refnum<queue>, error out=w660:errorcluster)  [unwired: 1 in, 1 out]
          }
        }
      }
      event "Right": Value Change {
        n296 = event-data() -> ()  [unwired: 1 in, 6 out]
        n297 = local read "Stanje"() -> (w667:string)
        n298 = call "Regular Timer Action Engine.vi"("Enum"=Control_Timer."Reset", "error in"=w662) -> ("error out"=w663:errorcluster)  [unwired: 7 in, 1 out]
        n299 = Equal?(x=w667, y="Ready") -> (x = y?=w665:bool)
        n300 = case shown="True" w665 {
          tunnel: w663 -> [w672 w680]
          tunnel: [w672 w675] -> w670
          tunnel: [w671 w674] -> w669
          tunnel: w668 -> [w671 w673]
          frame False {
          }
          frame True {
            n301 = shared-variable "RT CompactRIO Target\\Mod3\\DI8"(error in=w680) -> (w685:bool, error out=w679:errorcluster)
            n302 = shared-variable "RT CompactRIO Target\\Mod3\\DI10"(error in=w679) -> (w686:bool, error out=w678:errorcluster)
            n303 = shared-variable "RT CompactRIO Target\\Mod3\\DI12"(error in=w678) -> (w687:bool, error out=w677:errorcluster)
            n304 = shared-variable "RT CompactRIO Target\\Mod3\\DI13"(error in=w677) -> (w683:bool, error out=w676:errorcluster)
            n305 = Build Array(w685, w686, w687) -> (w684:bool[])
            n306 = And Array Elements(Boolean array=w684) -> (logical AND=w681:bool)
            n307 = Or(x=w681, y=w683) -> (x .or. y?=w682:bool)
            n308 = case shown="True" w682 {
              tunnel: w676 -> [w689 w694]
              tunnel: [w689 w699] -> w675
              tunnel: [w688 w698] -> w674
              tunnel: w673 -> [w688 w690]
              frame False {
              }
              frame True {
                n309 = shared-variable "RT CompactRIO Target\\Mod4\\DO12"(TRUE ("DO15"), error in=w694) -> (error out=w693:errorcluster)
                n310 = shared-variable "RT CompactRIO Target\\Mod4\\DO10"(TRUE ("DO13"), error in=w693) -> (error out=w692:errorcluster)
                n311 = shared-variable "RT CompactRIO Target\\Mod4\\DO9"(TRUE ("DO11"), error in=w692) -> (error out=w691:errorcluster)
                n312 = Enqueue Element(queue=w690, element="MoveRight", error in (no error)=w691) -> (queue out=w698:refnum<queue>, error out=w699:errorcluster)  [unwired: 1 in, 1 out]
              }
            }
          }
        }
      }
      event "Left": Value Change {
        n313 = event-data() -> ()  [unwired: 1 in, 6 out]
        n314 = local read "Stanje"() -> (w706:string)
        n315 = call "Regular Timer Action Engine.vi"("Enum"=Control_Timer."Reset", "error in"=w701) -> ("error out"=w702:errorcluster)  [unwired: 7 in, 1 out]
        n316 = Equal?(x=w706, y="Ready") -> (x = y?=w704:bool)
        n317 = case shown="True" w704 {
          tunnel: w702 -> [w711 w719]
          tunnel: [w711 w714] -> w709
          tunnel: [w710 w713] -> w708
          tunnel: w707 -> [w710 w712]
          frame False {
          }
          frame True {
            n318 = shared-variable "RT CompactRIO Target\\Mod3\\DI9"(error in=w719) -> (w724:bool, error out=w718:errorcluster)
            n319 = shared-variable "RT CompactRIO Target\\Mod3\\DI11"(error in=w718) -> (w725:bool, error out=w717:errorcluster)
            n320 = shared-variable "RT CompactRIO Target\\Mod3\\DI14"(error in=w717) -> (w726:bool, error out=w716:errorcluster)
            n321 = shared-variable "RT CompactRIO Target\\Mod3\\DI13"(error in=w716) -> (w722:bool, error out=w715:errorcluster)
            n322 = Build Array(w724, w725, w726) -> (w723:bool[])
            n323 = And Array Elements(Boolean array=w723) -> (logical AND=w720:bool)
            n324 = Or(x=w720, y=w722) -> (x .or. y?=w721:bool)
            n325 = case shown="True" w721 {
              tunnel: w715 -> [w728 w733]
              tunnel: [w728 w738] -> w714
              tunnel: [w727 w736] -> w713
              tunnel: w712 -> [w727 w737]
              frame False {
              }
              frame True {
                n326 = shared-variable "RT CompactRIO Target\\Mod4\\DO13"(TRUE ("DO15"), error in=w733) -> (error out=w732:errorcluster)
                n327 = shared-variable "RT CompactRIO Target\\Mod4\\DO11"(TRUE ("DO13"), error in=w732) -> (error out=w731:errorcluster)
                n328 = shared-variable "RT CompactRIO Target\\Mod4\\DO9"(FALSE ("DO9"), error in=w731) -> (error out=w730:errorcluster)
                n329 = Enqueue Element(queue=w737, element="MoveLeft", error in (no error)=w730) -> (queue out=w736:refnum<queue>, error out=w738:errorcluster)  [unwired: 1 in, 1 out]
              }
            }
          }
        }
      }
      event "Center": Value Change {
        n330 = event-data() -> ()  [unwired: 1 in, 6 out]
        n331 = local read "Stanje"() -> (w743:string)
        n332 = Equal?(x=w743, y="Ready") -> (x = y?=w744:bool)
        n333 = call "Regular Timer Action Engine.vi"("Enum"=Control_Timer."Reset", "error in"=w740) -> ("error out"=w742:errorcluster)  [unwired: 7 in, 1 out]
        n334 = case shown="True" w744 {
          tunnel: w742 -> [w750 w766]
          tunnel: [w750 w763] -> w748
          tunnel: [w749 w762] -> w747
          tunnel: w746 -> [w749 w761]
          frame False {
          }
          frame True {
            n335 = shared-variable "RT CompactRIO Target\\Mod3\\DI9"(error in=w766) -> (w770:bool, error out=w765:errorcluster)
            n336 = shared-variable "RT CompactRIO Target\\Mod3\\DI11"(error in=w765) -> (w771:bool, error out=w764:errorcluster)
            n337 = shared-variable "RT CompactRIO Target\\Mod3\\DI14"(error in=w764) -> (w751:bool, error out=w757:errorcluster)
            n338 = shared-variable "RT CompactRIO Target\\Mod3\\DI8"(error in=w757) -> (w759:bool, error out=w756:errorcluster)
            n339 = Build Array(w770, w771, w751) -> (w769:bool[])
            n340 = shared-variable "RT CompactRIO Target\\Mod3\\DI10"(error in=w756) -> (w760:bool, error out=w755:errorcluster)
            n341 = And Array Elements(Boolean array=w769) -> (logical AND=w767:bool)
            n342 = shared-variable "RT CompactRIO Target\\Mod3\\DI12"(error in=w755) -> (w752:bool, error out=w754:errorcluster)
            n343 = Build Array(w759, w760, w752) -> (w758:bool[])
            n344 = And Array Elements(Boolean array=w758) -> (logical AND=w753:bool)
            n345 = Or(x=w767, y=w753) -> (x .or. y?=w768:bool)
            n346 = case shown="True" w768 {
              tunnel: w754 -> [w773 w775]
              tunnel: [w773 w780] -> w763
              tunnel: [w772 w778] -> w762
              tunnel: w761 -> [w772 w779]
              tunnel: w752 -> [_ w777]
              tunnel: w751 -> [_ w776]
              frame False {
              }
              frame True {
                n347 = case shown="False" w777 {
                  tunnel: w776 -> [w784 _]
                  tunnel: w775 -> [w783 w790]
                  tunnel: [w782 w789] -> w774
                  frame False {
                    n348 = case shown="False" w784 {
                      tunnel: w783 -> [w785 w787]
                      tunnel: [w785 w786] -> w782
                      frame False {
                      }
                      frame True {
                        n349 = shared-variable "RT CompactRIO Target\\Mod4\\DO13"(TRUE ("DO15"), error in=w787) -> (error out=w786:errorcluster)
                      }
                    }
                  }
                  frame True {
                    n350 = shared-variable "RT CompactRIO Target\\Mod4\\DO12"(TRUE ("DO14"), error in=w790) -> (error out=w789:errorcluster)
                  }
                }
                n351 = Enqueue Element(queue=w779, element="MoveCenter", error in (no error)=w774) -> (queue out=w778:refnum<queue>, error out=w780:errorcluster)  [unwired: 1 in, 1 out]
              }
            }
          }
        }
      }
    }
    n352 = case shown="No Error" w578 {
      selector: w578 -> [w580 w584]
      tunnel: w577 -> [w581 w586]
      tunnel: [w581 w583] -> w576
      tunnel: [w580 w582] -> w574
      frame No Error {
      }
      frame Error {
        n353 = Enqueue Element(queue=w586, element="Shutdown") -> (queue out=w583:refnum<queue>, error out=w585:errorcluster)  [unwired: 2 in, 1 out]
        n354 = Merge Errors(w585, w584) -> (w582:errorcluster)
      }
    }
  }
  n355 = local read item#-1() -> ()  [unwired: 1 in]
  n356 = Merge Errors(w3, w4) -> (w2:errorcluster)
  n357 = Release Queue(queue=w6, error in (no error)=w2) -> (error out=→"error out":errorcluster)  [unwired: 1 in, 2 out]
